vi "Add or Remove Menu Items.vi"(8 "error in (no error)":errorcluster, 9 "Menu Items":T1[](array[typedef]), 10 "Menu in":refnum<k9>) -> (0 "error out":errorcluster, 2 "Menu out":refnum<k9>)   [LabVIEW 2016, in "Code String.lvclass"]
doc: "Adds/removes <b>Menu Items</b> from <b>Menu</b>.\n--------------------\nCopyright (c) 2019 Analog Devices, Inc. All rights reserved.\n\nRedistribution and use in source and binary forms, with or without modification,\nare permitted provided that the following conditions are met:\n - Redistributions of source code must retain the above copyright notice, this\n list of conditions and the following disclaimer.\n - Redistributions in binary form must reproduce the above copyright notice,\n this list of conditions and the following disclaimer in the documentation\n and/or other materials provided with the distribution.\n - Modified versions of the software must be conspicuously marked as such.\n - This software is licensed solely and exclusively for use with\n processors/products manufactured by or for Analog Devices, Inc.\n - This software may not be combined or merged with other code in any manner\n that would cause the software to become subject to terms and conditions\n which differ from those listed here.\n - Neither the name of Analog Devices, Inc. nor the names of its contributors\n may be used to endorse or promote products derived from this software\n without specific prior written permission.\n - The use of this software may or may not infringe the patent rights of one or\n more patent holders. This license does not release you from the requirement\n that you obtain separate licenses from these patent holders to use this\n software.\n\nTHIS SOFTWARE IS PROVIDED BY ANALOG DEVICES, INC. AND CONTRIBUTORS \"AS IS\" AND\nANY EXPRESS OR IMPLIED WARRANTIES, INCLUDING, BUT NOT LIMITED TO,\nNON-INFRINGEMENT, TITLE, MERCHANTABILITY AND FITNESS FOR A PARTICULAR PURPOSE\nARE DISCLAIMED. IN NO EVENT SHALL ANALOG DEVICES, INC. OR CONTRIBUTORS BE LIABLE\nFOR ANY DIRECT, INDIRECT, INCIDENTAL, SPECIAL, EXEMPLARY, PUNITIVE OR\nCONSEQUENTIAL DAMAGES (INCLUDING, BUT NOT LIMITED TO, DAMAGES ARISING OUT OF\nCLAIMS OF INTELLECTUAL PROPERTY RIGHTS INFRINGEMENT; PROCUREMENT OF SUBSTITUTE\nGOODS OR SERVICES; LOSS OF USE, DATA, OR PROFITS; OR BUSINESS INTERRUPTION)\nHOWEVER CAUSED AND ON ANY THEORY OF LIABILITY, WHETHER IN CONTRACT, STRICT\nLIABILITY, OR TORT (INCLUDING NEGLIGENCE OR OTHERWISE) ARISING IN ANY WAY OUT OF\nTHE USE OF THIS SOFTWARE, EVEN IF ADVISED OF THE POSSIBILITY OF SUCH DAMAGE.\n\n2019-01-10-7CBSD SLA"
uses:
  Code String.lvclass
  Events/Menu Item.ctl
panel:
  # "Copyright (c) 2019 Analog Devices, Inc.  All rights reserved.\n\nRedistribution and use in source and binary forms, with or without modification,\nare permitted provided that the following conditions are met:\n  - Redistributions of source code must retain the above copyright notice, this\n    list of conditions and the following disclaimer.\n  - Redistributions in binary form must reproduce the above copyright notice,\n    this list of conditions and the following disclaimer in the documentation\n    and/or other materials provided with the distribution.\n  - Modified versions of the software must be conspicuously marked as such.\n  - This software is licensed solely and exclusively for use with\n    processors/products manufactured by or for Analog Devices, Inc.\n  - This software may not be combined or merged with other code in any manner\n    that would cause the software to become subject to terms and conditions\n    which differ from those listed here.\n  - Neither the name of Analog Devices, Inc. nor the names of its contributors\n    may be used to endorse or promote products derived from this software\n    without specific prior written permission.\n  - The use of this software may or may not infringe the patent rights of one or\n    more patent holders.  This license does not release you from the requirement\n    that you obtain separate licenses from these patent holders to use this\n    software.\n\nTHIS SOFTWARE IS PROVIDED BY ANALOG DEVICES, INC. AND CONTRIBUTORS \"AS IS\" AND\nANY EXPRESS OR IMPLIED WARRANTIES, INCLUDING, BUT NOT LIMITED TO,\nNON-INFRINGEMENT, TITLE, MERCHANTABILITY AND FITNESS FOR A PARTICULAR PURPOSE\nARE DISCLAIMED. IN NO EVENT SHALL ANALOG DEVICES, INC. OR CONTRIBUTORS BE LIABLE\nFOR ANY DIRECT, INDIRECT, INCIDENTAL, SPECIAL, EXEMPLARY, PUNITIVE OR\nCONSEQUENTIAL DAMAGES (INCLUDING, BUT NOT LIMITED TO, DAMAGES ARISING OUT OF\nCLAIMS OF INTELLECTUAL PROPERTY RIGHTS INFRINGEMENT; PROCUREMENT OF SUBSTITUTE\nGOODS OR SERVICES; LOSS OF USE, DATA, OR PROFITS; OR BUSINESS INTERRUPTION)\nHOWEVER CAUSED AND ON ANY THEORY OF LIABILITY, WHETHER IN CONTRACT, STRICT\nLIABILITY, OR TORT (INCLUDING NEGLIGENCE OR OTHERWISE) ARISING IN ANY WAY OUT OF\nTHE USE OF THIS SOFTWARE, EVEN IF ADVISED OF THE POSSIBILITY OF SUCH DAMAGE.\n\n2019-01-10-7CBSD SLA"
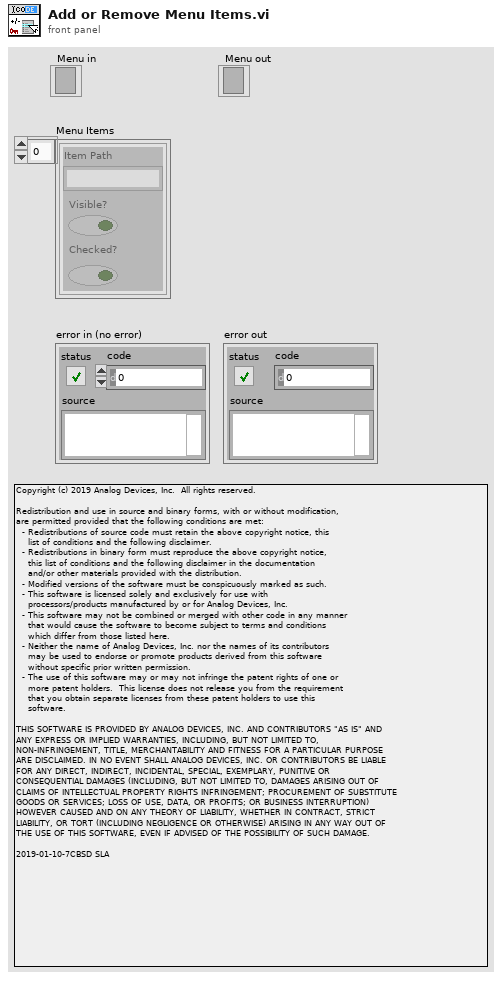
[diagram p1: front panel]
types:
  T1 = typedef "Code String.lvclass/Menu Item.ctl" = cluster{"Item Path":string, "Visible?":bool, "Checked?":bool}
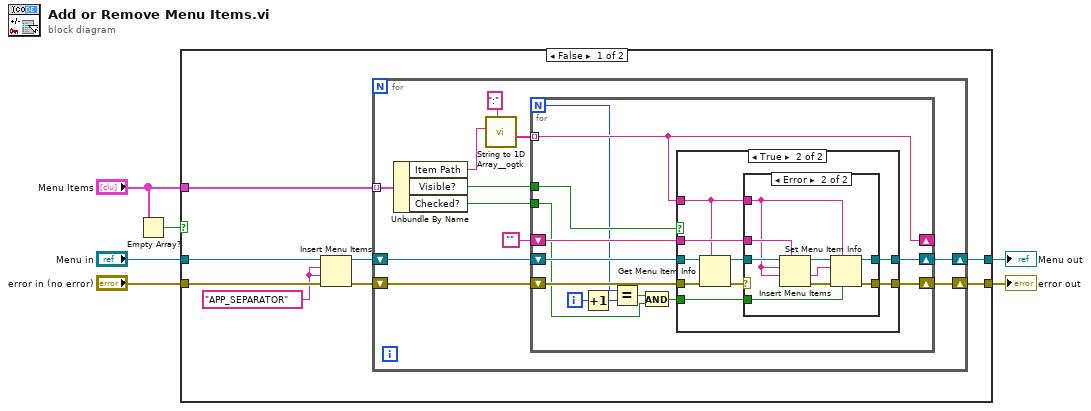
[diagram p0: block diagram]
diagram:
  n1 = Empty Array?(array="Menu Items") -> (empty?=w1:bool)
  n2 = case shown="False" w1 {
    tunnel: "error in (no error)" -> [w14 w62]
    tunnel: "Menu in" -> [w13 w61]
    tunnel: "Menu Items" -> [w11 _]
    tunnel: [w9 w62] -> w3
    tunnel: [w8 w61] -> w2
    frame False {
      w7 = "APP_SEPARATOR"
      n3 = Insert Menu Items(6:w14, 7:w7, 8:w7, 9:w13) -> (0:w10:errorcluster, 3:w12:refnum<k9>)  [unwired: 2 in, 1 out]
      n4 = for {
        shift-right: [w25] -> w8
        shift-left: w12 -> [w24]
        tunnel: w11 -> [w17] mode=indexing
        shift-right: [w15] -> w9
        shift-left: w10 -> [w16]
        n5 = Unbundle By Name(w17) -> ("Item Path"=w20:string, "Visible?"=w19:bool, "Checked?"=w18:bool)
        n6 = call <userlib>:"String to 1D Array__ogtk.vi"("delimiter (Tab)"=":", "string"=w20) -> ("Array of Strings"=w21:string[])  [unwired: 9 in]
        n7 = for {
          N -> [w29]
          shift-right: [w37] -> w25
          shift-left: w24 -> [w38]
          shift-right: [w32] -> _
          shift-left: "" -> [w36]
          tunnel: w21 -> [w32] mode=indexing
          tunnel: w19 -> [w35]
          tunnel: w18 -> [w27]
          shift-right: [w33] -> w15
          shift-left: w16 -> [w34]
          i -> [w31]
          n8 = Increment(x=w31) -> (x+1=w30:i32)
          n9 = Equal?(x=w29, y=w30) -> (x = y?=w28:bool)
          n10 = And(x=w28, y=w27) -> (x .and. y?=w26:bool)
          n11 = case shown="True" w35 {
            tunnel: w38 -> [w40 w49]
            tunnel: [w40 w44] -> w37
            tunnel: w36 -> [_ w46]
            tunnel: w32 -> [_ w45]
            tunnel: w26 -> [_ w43]
            tunnel: w34 -> [w39 w42]
            tunnel: [w39 w41] -> w33
            frame False {
            }
            frame True {
              n12 = Get Menu Item Info(7:w45, 8:w42, 11:w49) -> (0:w48:errorcluster, 3:w47:refnum<k9>)  [unwired: 5 out]
              n13 = case shown="Error" w48 {
                selector: w48 -> [w50 _]
                tunnel: w47 -> [w51 w60]
                tunnel: [w51 w57] -> w44
                tunnel: w46 -> [_ w59]
                tunnel: w45 -> [_ w53]
                tunnel: w43 -> [_ w56]
                tunnel: [w50 w54] -> w41
                frame No Error {
                }
                frame Error {
                  n14 = Insert Menu Items(5:w59, 7:w53, 8:w53, 9:w60) -> (0:w55:errorcluster, 1:w52:string, 3:w58:refnum<k9>)  [unwired: 2 in]
                  n15 = Set Menu Item Info(6:w56, 7:w53, 8:w55, 10:w52, 11:w58) -> (0:w54:errorcluster, 3:w57:refnum<k9>)  [unwired: 2 in]
                }
              }
            }
          }
        }
      }
    }
    frame True {
    }
  }
  "Menu out" <- w2
  "error out" <- w3
